vi "URAPI_Start_Subroutine.vi"(2 "Subroutine Name":string="Sub1", 3 "URAPI Script":T1) -> (1 "URAPI Script out":T1)   [LabVIEW 2012]
uses:
  <userlib>/BotSpeak/VIs/Direct/URAPI_Control.ctl
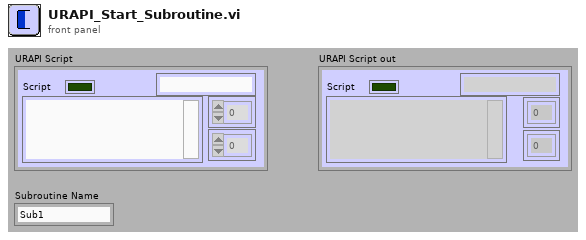
[diagram p1: front panel]
types:
  T1 = typedef "URAPI_Control.ctl" = cluster{"Script":string, "Whiles":u8[], "Ifs":u8[], "Supress Err":bool, "Errors":string}
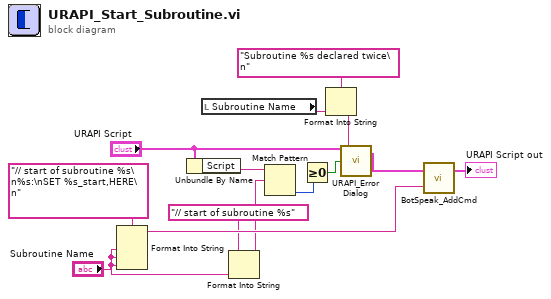
[diagram p0: block diagram]
diagram:
  n1 = Format Into String(format string="// start of subroutine %s\n%s:\nSET %s_start,HERE\n" ("String"), "Subroutine Name", "Subroutine Name", "Subroutine Name") -> (resulting string=w14:string)  [unwired: 2 in, 1 out]
  n2 = Unbundle By Name("URAPI Script") -> ("Script"=w11:string)
  n3 = local read "Subroutine Name"() -> (w3:string)
  n4 = Format Into String(format string="// start of subroutine %s" ("String"), "Subroutine Name") -> (resulting string=w5:string)  [unwired: 2 in, 1 out]
  n5 = Match Pattern(string=w11, regular expression=w5) -> (offset past match=w10:i32)  [unwired: 1 in, 3 out]
  n6 = Greater Or Equal To 0?(x=w10) -> (x >= 0?=w9:bool)
  n7 = Format Into String(format string="Subroutine %s declared twice\n" ("Error String"), w3) -> (resulting string=w2:string)  [unwired: 2 in, 1 out]
  n8 = call <userlib>:"URAPI_Error Dialog.vi"("Error String"=w2, "Error?"=w9, "URAPI Script in"="URAPI Script") -> ("URAPI Script out"=w7:T1)  [unwired: 1 in]
  n9 = call <userlib>:"BotSpeak_AddCmd.vi"("String"=w14, "URAPI Script"=w7) -> ("URAPI Script out"=→"URAPI Script out":T1)  [unwired: 1 in]
